vi "ASK.vi"() -> ()   [LabVIEW 2014]
uses:
  <vilib>/Analysis/8numeric.llb/1D Numeric Integration.vi
  <vilib>/Analysis/NI_AALPro.lvlib
panel:
  out "Demod Waveform":i16[](graph)
  out "Waveform Chart":dbl[](graph)
  out "ASK mod Waveform":dbl[](graph)
  out "Carrier Waveform":dbl[](graph)
  out "Input Waveform":i16[](graph)
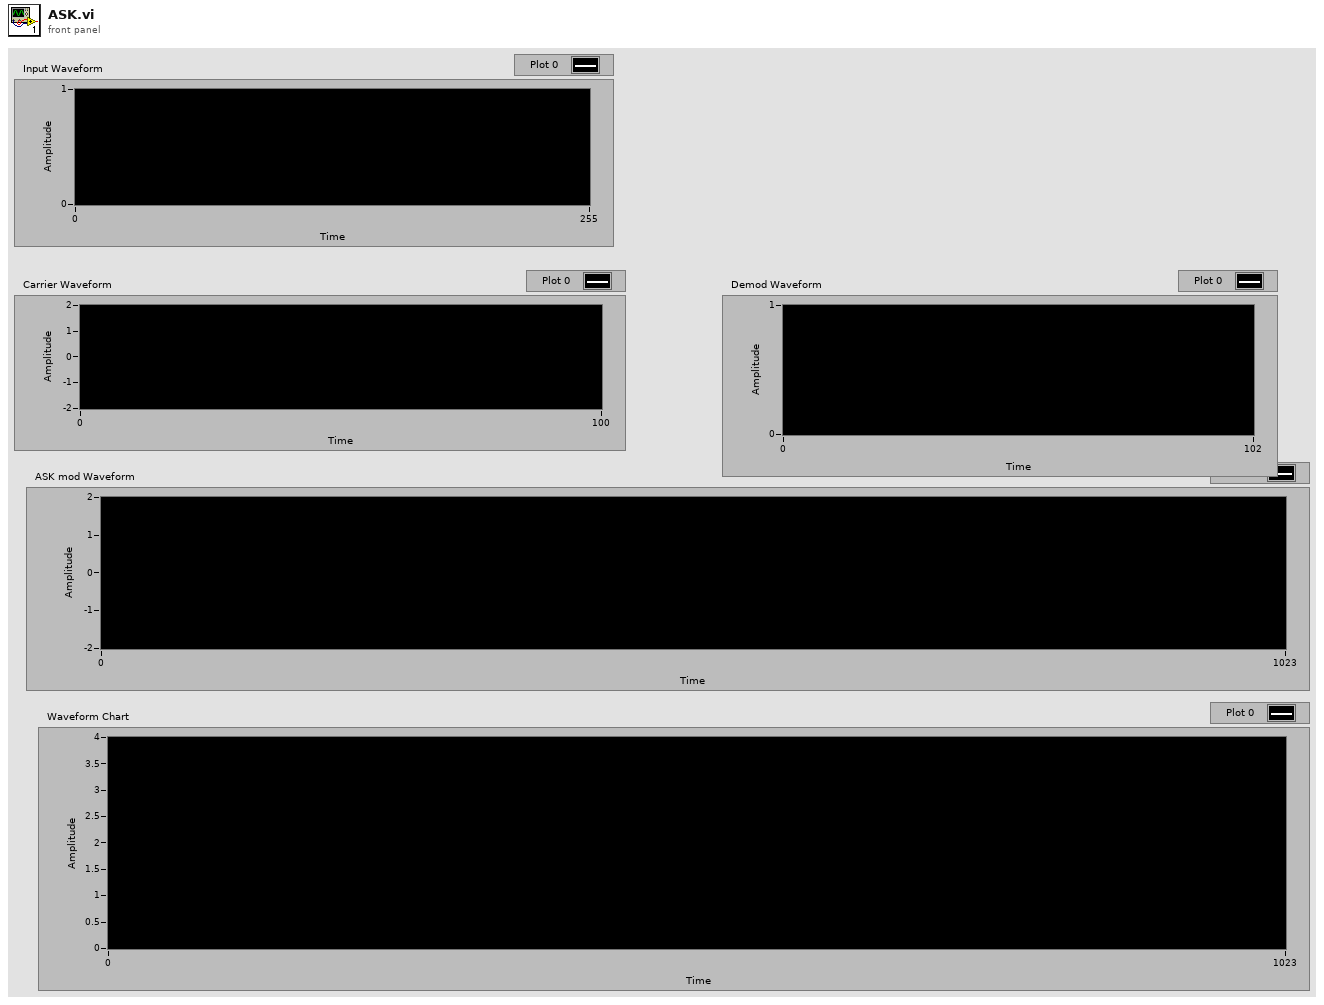
[diagram p1: front panel]
types:
  T1 = enum16{"sine", "cosine", "triangle", "square", "sawtooth", "increasing ramp", "decreasing ramp"}
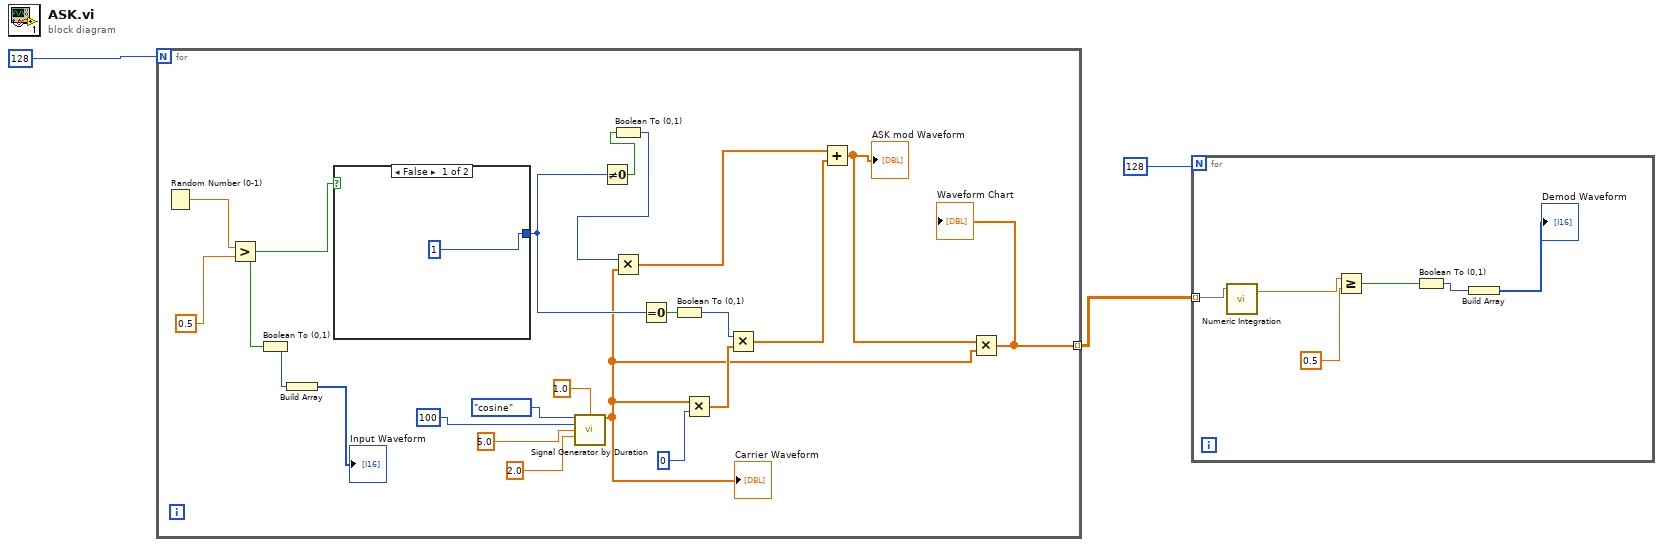
[diagram p0: block diagram]
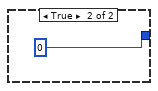
[diagram p2: hidden frame]
diagram:
  n1 = for {
    N: 128 -> [_]
    tunnel: [w4] -> w2 mode=indexing
    n2 = Random Number (0-1)() -> (number: 0 to 1=w25:dbl)
    n3 = Greater?(x=w25, y=0.5) -> (0:w23:bool)
    n4 = Boolean To (0,1)(Boolean=w23) -> (0, 1=w22:i16)
    n5 = Build Array(w22) -> (→"Input Waveform":i16[])
    n6 = case shown="False" w23 {
      tunnel: [1 0] -> w14
      frame False {
      }
      frame True {
      }
    }
    n7 = call <vilib>:"Signal Generator by Duration.vi"("signal type"=T1."cosine", "duration"=1.0, "# of samples"=100, "frequency"=5.0, "amplitude"=2.0) -> ("signal"=w5:dbl[])  [unwired: 7 in, 3 out]
    "Carrier Waveform" <- w5
    n8 = Not Equal To 0?(x=w14) -> (x != 0?=w16:bool)
    n9 = Boolean To (0,1)(Boolean=w16) -> (0, 1=w15:i16)
    n10 = Multiply(x=w15, y=w5) -> (x*y=w9:dbl[])
    n11 = Equal To 0?(x=w14) -> (x = 0?=w13:bool)
    n12 = Boolean To (0,1)(Boolean=w13) -> (0, 1=w11:i16)
    n13 = Multiply(x=w5, y=0) -> (x*y=w12:dbl[])
    n14 = Multiply(x=w11, y=w12) -> (x*y=w8:dbl[])
    n15 = Add(x=w9, y=w8) -> (x+y=w6:dbl[])
    "ASK mod Waveform" <- w6
    n16 = Multiply(x=w6, y=w5) -> (x*y=w4:dbl[])
    "Waveform Chart" <- w4
  }
  n17 = for {
    N: 128 -> [_]
    tunnel: w2 -> [w28] mode=indexing
    n18 = call-poly <vilib>:"Numeric Integration.vi"("Input Array"=w28) -> ("result"=w33:dbl)  [unwired: 2 in, 1 out]
    n19 = Greater Or Equal?(x=w33, y=0.5) -> (x >= y?=w31:bool)
    n20 = Boolean To (0,1)(Boolean=w31) -> (0, 1=w30:i16)
    n21 = Build Array(w30) -> (→"Demod Waveform":i16[])
  }
